vi "OBDservice06GetSupportMID.vi"(8 "error in (no error) 2":errorcluster, 11 "diag ref in":T1={"Diag CAN Handle"=0, "Transport Protocol"=enum."ISO TP - Normal Mode", "Receive Address Extension"=0, "Transmit Address Extension"=0, "Receive CAN Id"=0, "Transmit CAN Id"=0, "Log Frames ?"=FALSE, "My TP Address"=0, "Other TP Address"=0, "T1"=0, "T2"=0, "T3"=0, "T4"=0, "Tx SN"=0, "Block Size"=0, "Rx SN"=0, "VW TP Initialized?"=FALSE, "Tx block no"=0, "baud rate"=0, "Interface"="", "Channel Diag CAN Handle"=0, "UDP Connection ID"=refnum, "TCP Connection ID"=refnum, "Target IP Addr"=0, "Source Address"=0, "Target Address"=0, "Send Header NACK?"=FALSE, "DLL Handle"=0, "NAD"=0, "Time Stamp read first"=0.0, "Time Stamp read last"=0.0, "Time Stamp write first"=0.0, "Time Stamp write last"=0.0, "Time Stamp write"=0.0, "Time Stamp read"=0.0, " I/O Mode"=0, "FD Baudrate"=0, "TX_DL"=8, "RX_DL"=8, "DoIP Protocol Version"=1, " Selected I/O Mode"=0, "TesterPresent Counter"=0, "TesterPresent Limit"=0, "TesterPresent Tick[ms]"=10, "TesterPresent RequireResponse?"=FALSE, "TesterPresent Stored Ref?"=FALSE, "TesterPresent Message"=[], "TesterPresent Task Handle"=0, "TesterPresent Semaphore"=refnum, "Response Plausibility Check"=1, "Default Version?"=TRUE, "Diagostic Globals"={"Timeout FC (Bs)"=250, "Timeout CF (Cr)"=250, "Timeout Diag Command"=1000, "Receive Block Size (BS)"=0, "Wait Time CF (STmin)"=5, "Max Waits (N_WFTmax)"=10, "Waits to Send (N_WAIT)"=0, "Time between Waits (TW)"=25, "Fill CAN Frames?"=TRUE, "Fill Byte"=255, "Invalid Response as Error?"=FALSE, "Max RspPending Count"=5, "VWTP Command Timeout"=50, "Transport Protocol"=enum."Diagnostics on IP", "Diag CAN Handle"=0, "DLL Handle"=0, "Timeout RspPending"=1000}, "Session-based Properties?"=FALSE} {"Diagostic Globals"."Fill Byte" format="%x"; "TesterPresent Message" format="%.0x"; "Selected I/O Mode" items=["CAN", "CAN FD", "CAN FD+BRS", "ECU Determined"]; "DoIP Protocol Version" items=["2010"=1, "2012"=2]; "RX_DL" items=["8"=8, "12"=12, "16"=16, "20"=20, "24"=24, "32"=32, "48"=48, "64"=64]; "TX_DL" items=["8"=8, "12"=12, "16"=16, "20"=20, "24"=24, "32"=32, "48"=48, "64"=64]; "I/O Mode" items=["CAN", "CAN FD", "CAN FD+BRS", "Not yet determined"]}) -> (0 "error out 2":errorcluster, 1 "success?":bool, 2 "MIDs out":u8[](array[numeric]), 3 "diag ref out 2":T1={"Diag CAN Handle"=0, "Transport Protocol"=enum."ISO TP - Normal Mode", "Receive Address Extension"=0, "Transmit Address Extension"=0, "Receive CAN Id"=0, "Transmit CAN Id"=0, "Log Frames ?"=FALSE, "My TP Address"=0, "Other TP Address"=0, "T1"=0, "T2"=0, "T3"=0, "T4"=0, "Tx SN"=0, "Block Size"=0, "Rx SN"=0, "VW TP Initialized?"=FALSE, "Tx block no"=0, "baud rate"=0, "Interface"="", "Channel Diag CAN Handle"=0, "UDP Connection ID"=refnum, "TCP Connection ID"=refnum, "Target IP Addr"=0, "Source Address"=0, "Target Address"=0, "Send Header NACK?"=FALSE, "DLL Handle"=0, "NAD"=0, "Time Stamp read first"=0.0, "Time Stamp read last"=0.0, "Time Stamp write first"=0.0, "Time Stamp write last"=0.0, "Time Stamp write"=0.0, "Time Stamp read"=0.0, " I/O Mode"=0, "FD Baudrate"=0, "TX_DL"=8, "RX_DL"=8, "DoIP Protocol Version"=1, " Selected I/O Mode"=0, "TesterPresent Counter"=0, "TesterPresent Limit"=0, "TesterPresent Tick[ms]"=10, "TesterPresent RequireResponse?"=FALSE, "TesterPresent Stored Ref?"=FALSE, "TesterPresent Message"=[], "TesterPresent Task Handle"=0, "TesterPresent Semaphore"=refnum, "Response Plausibility Check"=1, "Default Version?"=TRUE, "Diagostic Globals"={"Timeout FC (Bs)"=250, "Timeout CF (Cr)"=250, "Timeout Diag Command"=1000, "Receive Block Size (BS)"=0, "Wait Time CF (STmin)"=5, "Max Waits (N_WFTmax)"=10, "Waits to Send (N_WAIT)"=0, "Time between Waits (TW)"=25, "Fill CAN Frames?"=TRUE, "Fill Byte"=255, "Invalid Response as Error?"=FALSE, "Max RspPending Count"=5, "VWTP Command Timeout"=50, "Transport Protocol"=enum."Diagnostics on IP", "Diag CAN Handle"=0, "DLL Handle"=0, "Timeout RspPending"=1000}, "Session-based Properties?"=FALSE} {"Diagostic Globals"."Fill Byte" format="%x"; "TesterPresent Message" format="%.0x"; "Selected I/O Mode" items=["CAN", "CAN FD", "CAN FD+BRS", "ECU Determined"]; "DoIP Protocol Version" items=["2010"=1, "2012"=2]; "RX_DL" items=["8"=8, "12"=12, "16"=16, "20"=20, "24"=24, "32"=32, "48"=48, "64"=64]; "TX_DL" items=["8"=8, "12"=12, "16"=16, "20"=20, "24"=24, "32"=32, "48"=48, "64"=64]; "I/O Mode" items=["CAN", "CAN FD", "CAN FD+BRS", "Not yet determined"]})   [LabVIEW 2018]
uses:
  <vilib>/Automotive Diagnostic Command Set/Diagnostic Transport.llb/Diag Reference.ctl
  <vilib>/Automotive Diagnostic Command Set/Diagnostic Transport.llb/Transport Protocol Selector.ctl
  <vilib>/Automotive Diagnostic Command Set/Diagnostic Transport.llb/DoIP Protocol Version.ctl
  <vilib>/Automotive Diagnostic Command Set/Diagnostic Transport.llb/Diag Globals.ctl
  <vilib>/addons/Automotive Diagnostic Command Set/NI_Automotive Diagnostic Command Set.lvlib
panel:
  out "data out":u8[][](array[numeric]) format="%.0x"
  # "4"
  # "5"
  # "1"
  # "3"
  # "6"
  # "2"
  # "7"
  # "8"
  # "TID(转换方法)||DASID||TestValue high byte||TestValue low byte||MinTestLimit high byte||MinTestLimit low byte|||MaxTestLimit high byte||MaxTestLimit low byte||"
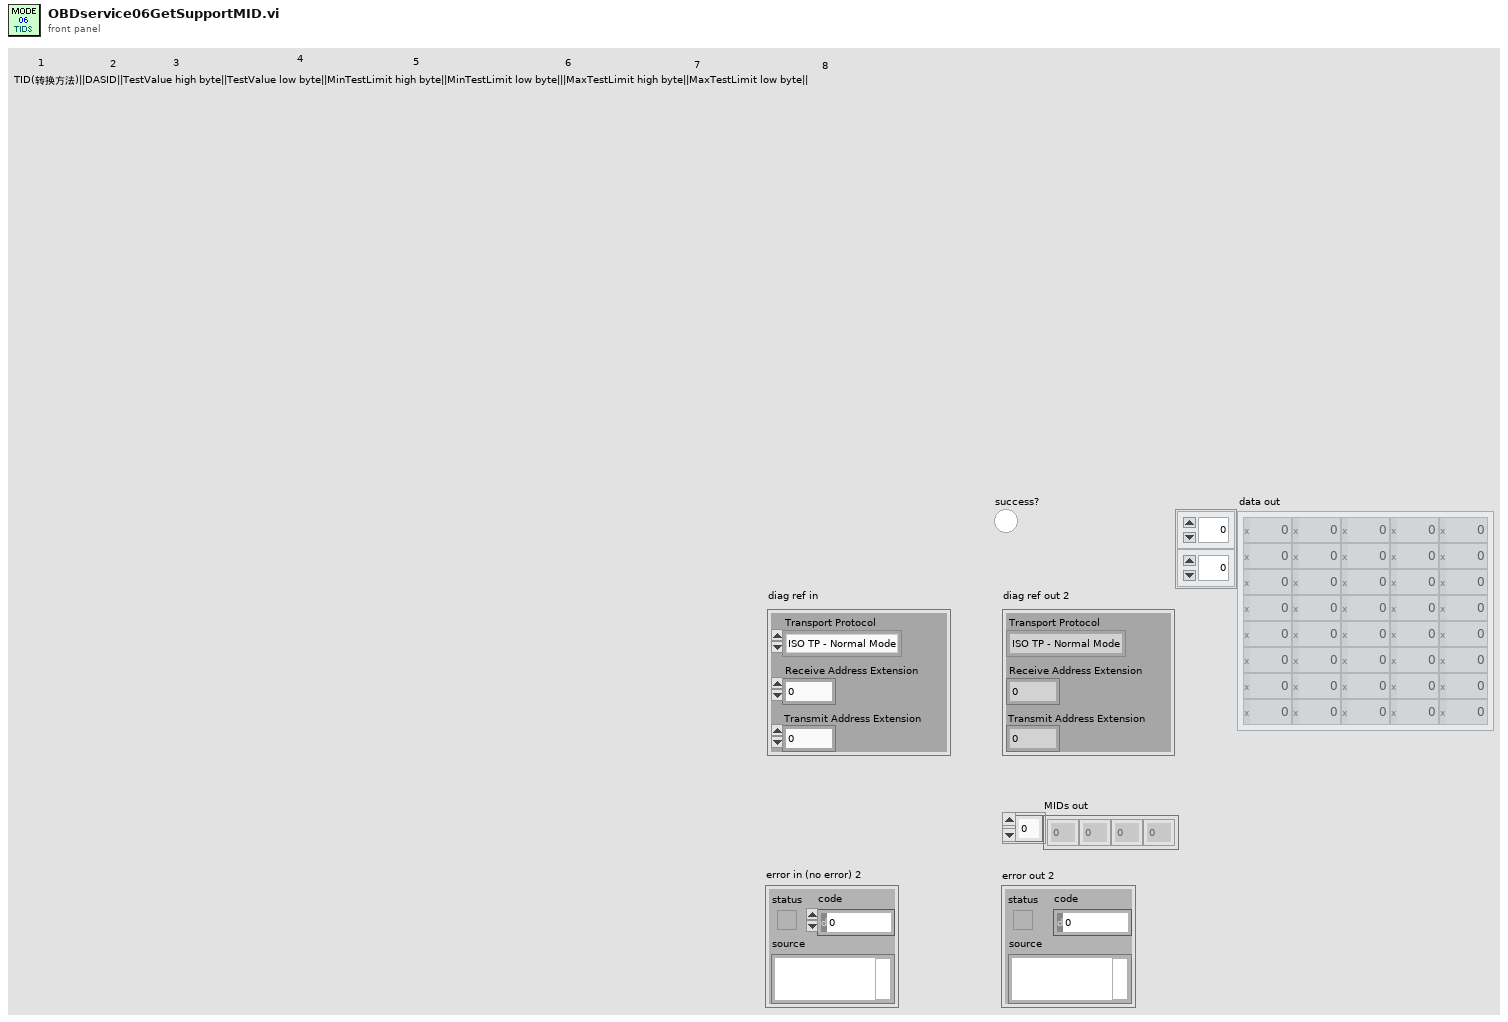
[diagram p1: front panel]
types:
  T1 = typedef "NI_Automotive Diagnostic Command Set.lvlib/Diag Reference.ctl" = cluster{"Diag CAN Handle":u32, "Transport Protocol":T2, "Receive Address Extension":u8, "Transmit Address Extension":u8, "Receive CAN Id":u32, "Transmit CAN Id":u32, "Log Frames ?":bool, "My TP Address":u8, "Other TP Address":u8, "T1":u16, "T2":u16, "T3":u16, "T4":u16, "Tx SN":u8, "Block Size":u8, "Rx SN":u8, "VW TP Initialized?":bool, "Tx block no":u8, "baud rate":u64, "Interface":string, "Channel Diag CAN Handle":u32, "UDP Connection ID":refnum<k16>, "TCP Connection ID":refnum<k5>, "Target IP Addr":u32, "Source Address":u16, "Target Address":u16, "Send Header NACK?":bool, "DLL Handle":u32, "NAD":u8, "Time Stamp read first":dbl, "Time Stamp read last":dbl, "Time Stamp write first":dbl, "Time Stamp write last":dbl, "Time Stamp write":dbl, "Time Stamp read":dbl, " I/O Mode":u32, "FD Baudrate":u64, "TX_DL":u16, "RX_DL":u16, "DoIP Protocol Version":T3, " Selected I/O Mode":u32, "TesterPresent Counter":u32, "TesterPresent Limit":u32, "TesterPresent Tick[ms]":i32, "TesterPresent RequireResponse?":bool, "TesterPresent Stored Ref?":bool, "TesterPresent Message":u8[], "TesterPresent Task Handle":i32, "TesterPresent Semaphore":T4, "Response Plausibility Check":u32, "Default Version?":bool, "Diagostic Globals":T5, "Session-based Properties?":bool}
  T2 = typedef "NI_Automotive Diagnostic Command Set.lvlib/Transport Protocol Selector.ctl" = enum16{"ISO TP - Normal Mode", "ISO TP - Mixed Mode", "VW TP 2.0", "Diagnostics on IP", "ISO TP LIN"}
  T3 = typedef "NI_Automotive Diagnostic Command Set.lvlib/DoIP Protocol Version.ctl" = u8
  T4 = typedef "Semaphore RefNum" = refnum<k1>
  T5 = typedef "NI_Automotive Diagnostic Command Set.lvlib/Diag Globals.ctl" = cluster{"Timeout FC (Bs)":u32, "Timeout CF (Cr)":u32, "Timeout Diag Command":u32, "Receive Block Size (BS)":u8, "Wait Time CF (STmin)":u8, "Max Waits (N_WFTmax)":u8, "Waits to Send (N_WAIT)":i32, "Time between Waits (TW)":u32, "Fill CAN Frames?":bool, "Fill Byte":u32, "Invalid Response as Error?":bool, "Max RspPending Count":u32, "VWTP Command Timeout":u32, "Transport Protocol":T2, "Diag CAN Handle":u32, "DLL Handle":u32, "Timeout RspPending":u32}
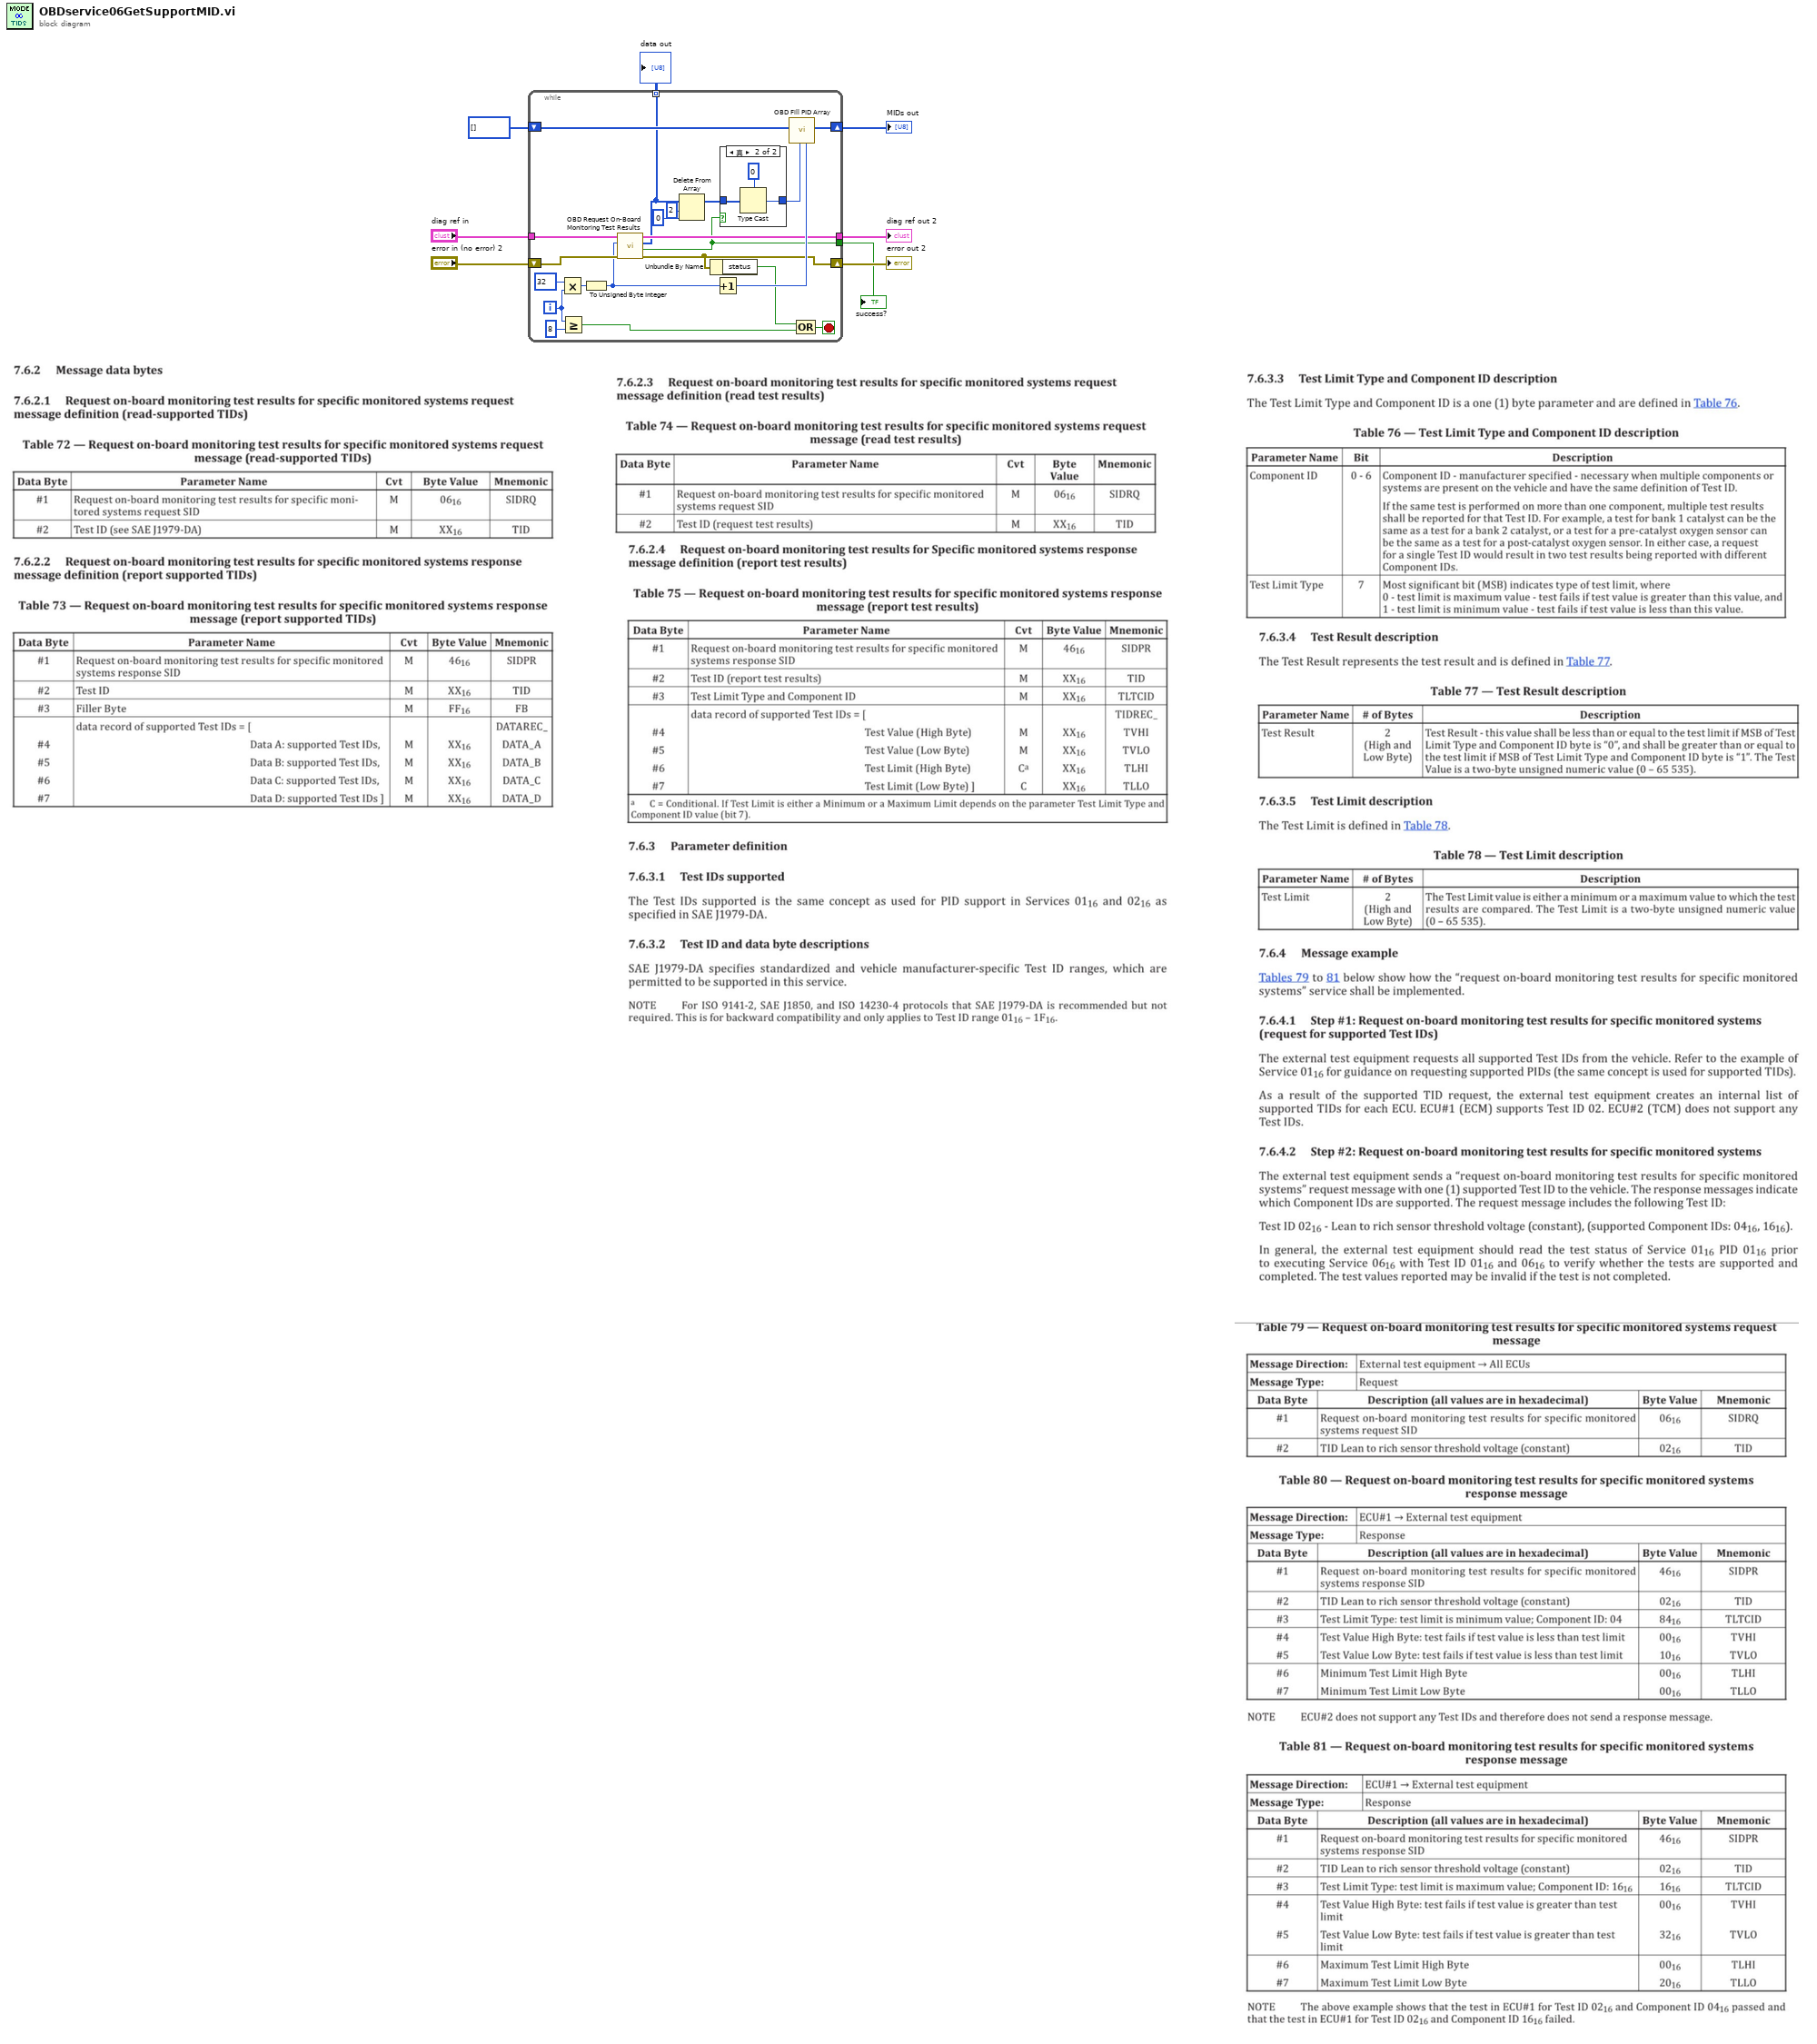
[diagram p0: block diagram]
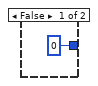
[diagram p2: hidden frame]
diagram:
  n1 = while {
    tunnel: "diag ref in" -> [w18]
    tunnel: [w15] -> w6
    shift-right: [w27] -> w3
    shift-left: u8[] [] -> [w28]
    shift-right: [w14] -> w5
    shift-left: "error in (no error) 2" -> [w17]
    tunnel: [w13] -> w2
    tunnel: [w9] -> w1 mode=indexing
    i -> [w23]
    stop <- w21 stop-if-true
    n2 = Multiply(x=32, y=w23) -> (x*y=w24:i32)
    n3 = Greater Or Equal?(x=w23, y=8) -> (x >= y?=w20:bool)
    n4 = To Unsigned Byte Integer(number=w24) -> (unsigned 8bit integer=w16:u8)
    n5 = call <vilib>:"OBD Request On-Board Monitoring Test Results.vi"("error in (no error)"=w17, "OBDMID"=w16, "diag ref in"=w18) -> ("error out"=w14:errorcluster, "success?"=w13:bool, "data out"=w9:u8[], "diag ref out"=w15:T1)  [unwired: 5 in]
    n6 = Delete From Array(array=w9, length=2 ("长度"), index=0 ("索引")) -> (array with subset deleted=w12:u8[])  [unwired: 1 out]
    n7 = Unbundle By Name(w14) -> ("status"=w19:bool)
    n8 = Increment(x=w16) -> (x+1=w25:u8)
    n9 = case shown="真" w13 {
      tunnel: w12 -> [_ w33]
      tunnel: [u32 0 w31] -> w26
      frame False {
      }
      frame True {
        n10 = Type Cast(type=u32 0, x=w33) -> (*(type *) &x=w31:u32)
      }
    }
    n11 = call <vilib>:"OBD Fill PID Array.vi"("first index"=w25, "bitfield"=w26, "PIDs in"=w28) -> ("PIDs out"=w27:u8[])  [unwired: 8 out]
    n12 = Compound Arithmetic op=OR(w19, w20) -> (w21:bool)
  }
  "error out 2" <- w5
  "MIDs out" <- w3
  "diag ref out 2" <- w6
  "success?" <- w2
  "data out" <- w1
